vi "Climber_Execute.vi"() -> ()   [LabVIEW 2020]
uses:
  Globals/Climber_Globals.vi
  <vilib>/Rock Robotics/WPI/Solenoid/WPI_SolenoidValue.ctl
panel:
  in  "Outer_Arm_Elevator_Lower_Limit":dbl
  in  "Outer_Arm_Elevator_Upper_Limit":dbl
  in  "Inner_Arm_Pivot_Lower_Limit":dbl
  in  "Inner_Arm_Pivot_Upper_Limit":dbl
  in  "Outer_Arm_Pivot_Lower_Limit":dbl
  in  "Outer_Arm_Pivot_Upper_Limit":dbl
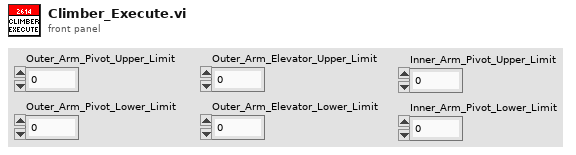
[diagram p1: front panel]
types:
  T1 = typedef "WPI_SolenoidValue.ctl" = enum16{"Off", "On", "Forward", "Reverse"}
  T2 = typedef "Climber_Cluster.ctl" = cluster{"Control_State":T3, "Outer_Arm_Pivot_Throttle":dbl, "Outer_Arm_Elevator_Throttle":dbl, "Inner_Arm_Pivot_Throttle":dbl, "Enable_Climber_Sequence":bool}
  T3 = typedef "Climber_Control_States.ctl" = enum16{"No-Op", "Manual_%Vbus", "Climbing_Sequence"}
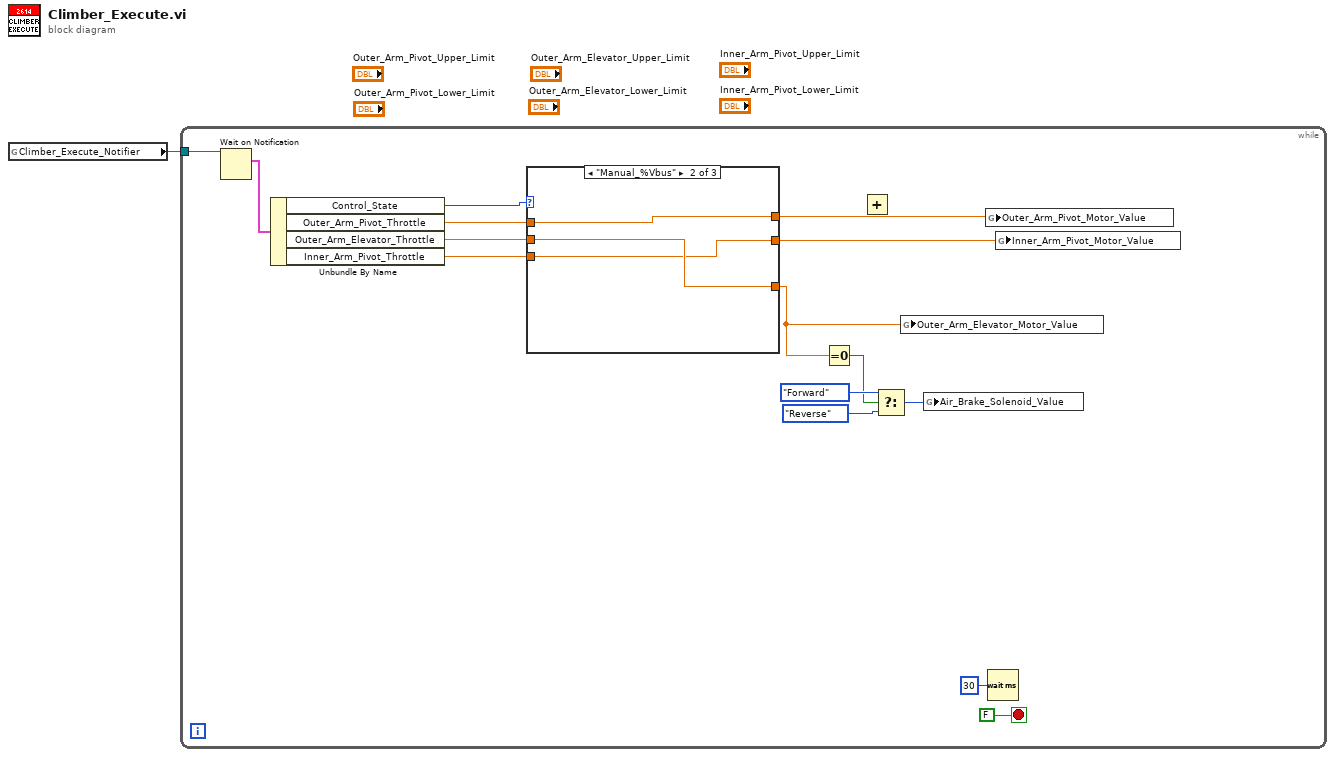
[diagram p0: block diagram]
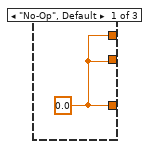
[diagram p2: hidden frame]
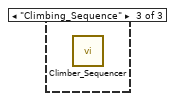
[diagram p3: hidden frame]
diagram:
  n1 = global read "Climber_Globals.vi" "Climber_Execute_Notifier"() -> (w1:refnum<notifier>)
  n2 = while {
    tunnel: w1 -> [w16]
    stop <- FALSE stop-if-true
    n3 = Wait on Notification(notifier=w16) -> (notification=w13:T2)  [unwired: 3 in, 3 out]
    n4 = Unbundle By Name(w13) -> ("Control_State"=w12:T3, "Outer_Arm_Pivot_Throttle"=w6:dbl, "Outer_Arm_Elevator_Throttle"=w5:dbl, "Inner_Arm_Pivot_Throttle"=w4:dbl)
    n5 = case shown="\"Manual_%Vbus\"" w12 {
      tunnel: [w17 w19 _] -> w11
      tunnel: [w17 w18 _] -> w2
      tunnel: [w17 w20 _] -> w3
      tunnel: w6 -> [_ w20 _]
      tunnel: w5 -> [_ w19 _]
      tunnel: w4 -> [_ w18 _]
      frame "No-Op", Default {
        w17 = 0.0 ("Outer_Arm_Elevator_Motor_Value")
      }
      frame "Manual_%Vbus" {
      }
      frame "Climbing_Sequence" {
        n6 = call "Climber_Sequencer.vi"() -> ()  [unwired: 4 in, 3 out]
      }
    }
    n7 = Equal To 0?(x=w11) -> (x = 0?=w8:bool)
    n8 = Add() -> ()  [unwired: 2 in, 1 out]
    n9 = Select(t=WPI_SolenoidValue."Forward" ("Air_Brake_Solenoid_Value"), s=w8, f=WPI_SolenoidValue."Reverse" ("Air_Brake_Solenoid_Value")) -> (s? t:f=w7:T1)
    n10 = global write "Climber_Globals.vi" "Outer_Arm_Elevator_Motor_Value"(w11) -> ()
    n11 = global write "Climber_Globals.vi" "Air_Brake_Solenoid_Value"(w7) -> ()
    n12 = global write "Climber_Globals.vi" "Outer_Arm_Pivot_Motor_Value"(w3) -> ()
    n13 = Wait (ms)(milliseconds to wait=u32 30) -> ()  [unwired: 1 out]
    n14 = global write "Climber_Globals.vi" "Inner_Arm_Pivot_Motor_Value"(w2) -> ()
  }
